vi "Read View VI and FP Refs.vi"(0 "GUI Container Actor in":refnum<class "GUI Container Actor.lvclass">, 5 "View":string, 7 "View Hierarchy Level":i32, 11 "error in (no error)":errorcluster) -> (4 "GUI Container Actor out":refnum<class "GUI Container Actor.lvclass">, 6 "View Status":T1, 8 "VI References":T4, 10 "View Found":bool, 15 "error out":errorcluster)   [LabVIEW 2023, in "GUI Views.lvlib" / "GUI Container Actor.lvclass"]
uses:
  GUI Container Actor.lvclass
  typedefs/VI References.ctl
  typedefs/View Status.ctl
  <vilib>/ActorFramework/Message Enqueuer/Message Enqueuer.lvclass
  typedefs/View Details.ctl
  typedefs/FP Status.ctl
  <userlib>/_OpenG.lib/error/error.llb/openg_error.lvlib
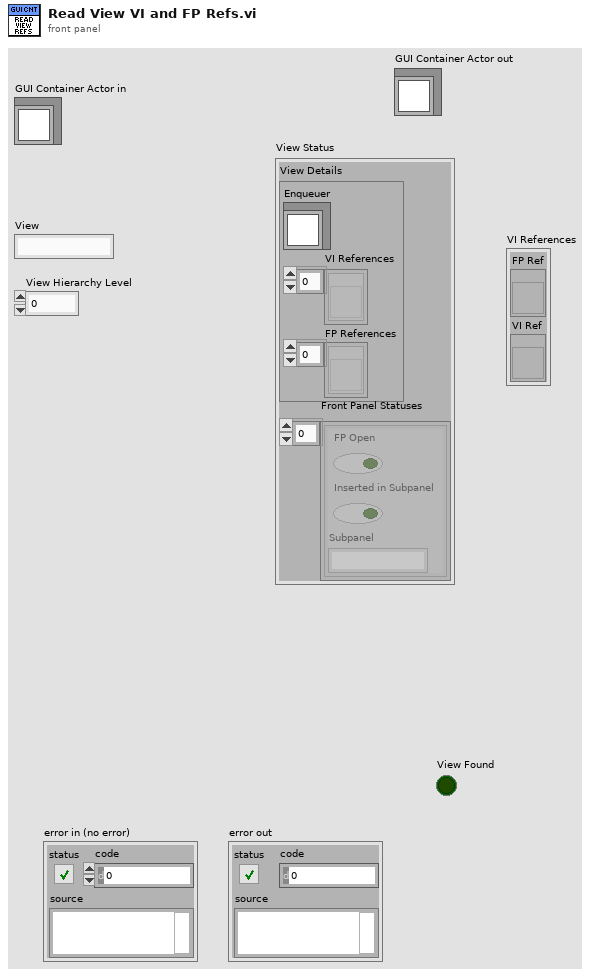
[diagram p1: front panel]
types:
  T1 = typedef "GUI Views.lvlib/GUI Container Actor.lvclass/View Status.ctl" = cluster{"View Details":T2, "Front Panel Statuses":T3[]}
  T2 = typedef "GUI Views.lvlib/GUI Container Actor.lvclass/View Details.ctl" = cluster{"Enqueuer":refnum<class "Message Enqueuer.lvclass">, "VI References":refnum<vi>[], "FP References":refnum<vi>[]}
  T3 = typedef "GUI Views.lvlib/GUI Container Actor.lvclass/FP Status.ctl" = cluster{"FP Open":bool, "Inserted in Subpanel":bool, "Subpanel":string}
  T4 = typedef "GUI Views.lvlib/GUI Container Actor.lvclass/VI References.ctl" = cluster{"FP Ref":refnum<vi>, "VI Ref":refnum<vi>}
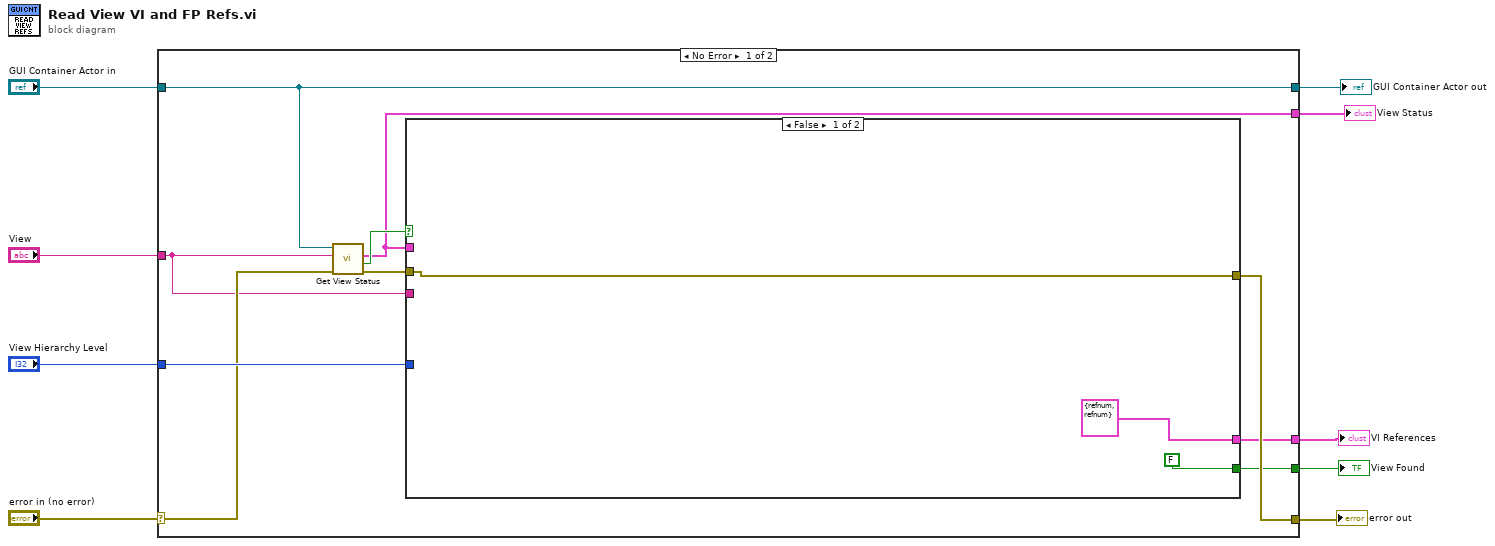
[diagram p0: block diagram]
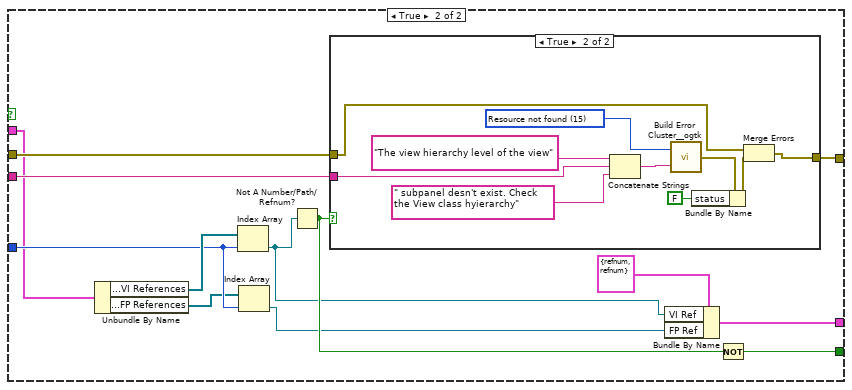
[diagram p2: hidden frame]
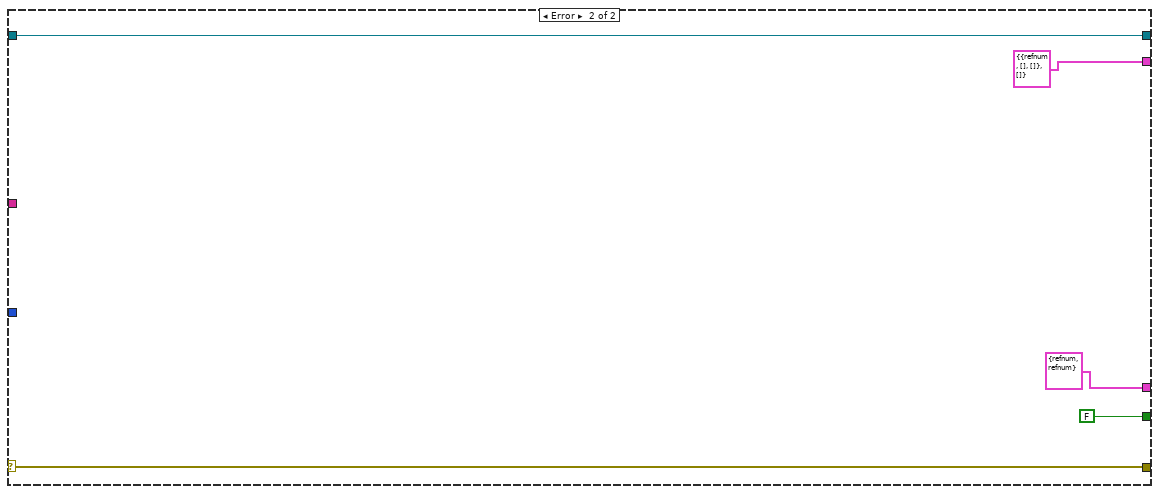
[diagram p4: hidden frame]
diagram:
  n1 = case shown="No Error" "error in (no error)" {
    selector: "error in (no error)" -> [w16 w50]
    tunnel: [w19 w50] -> w9
    tunnel: "GUI Container Actor in" -> [w13 w51]
    tunnel: "View Hierarchy Level" -> [w18 _]
    tunnel: "View" -> [w14 _]
    tunnel: [w13 w51] -> w4
    tunnel: [w17 FALSE] -> w3
    tunnel: [w11 T4 {"FP Ref"=refnum, "VI Ref"=refnum} ("VI References")] -> w2
    tunnel: [w10 T1 {"View Details"={"Enqueuer"=refnum, "VI References"=[], "FP References"=[]}, "Front Panel Statuses"=[]} ("View State")] -> w1
    frame No Error {
      n2 = call "Get View Status.vi"("error in (no error)"=w16, "View"=w14, "GUI Container View Actor in"=w13) -> ("error out"=w15:errorcluster, "View Found"=w12:bool, "View Status"=w10:T1)  [unwired: 5 in, 1 out]
      n3 = case shown="False" w12 {
        tunnel: w15 -> [w22 w34]
        tunnel: w18 -> [_ w32]
        tunnel: [w22 w33] -> w19
        tunnel: w14 -> [_ w31]
        tunnel: [FALSE w23] -> w17
        tunnel: w10 -> [_ w28]
        tunnel: [T4 {"FP Ref"=refnum, "VI Ref"=refnum} ("VI References") w24] -> w11
        frame False {
        }
        frame True {
          n4 = Unbundle By Name(w28) -> ("View Details.VI References"=w35:refnum<vi>[], "View Details.FP References"=w30:refnum<vi>[])
          n5 = Index Array(array=w35, index=w32) -> (element=w25:refnum<vi>)
          n6 = Index Array(array=w30, index=w32) -> (element=w26:refnum<vi>)
          n7 = Not A Number/Path/Refnum?(number/path/refnum=w25) -> (NaN/Path/Refnum?=w29:bool)
          n8 = case shown="True" w29 {
            tunnel: w34 -> [w36 w42]
            tunnel: [w36 w40] -> w33
            tunnel: w31 -> [_ w39]
            frame False {
            }
            frame True {
              w43 = 15 items=["No error", "Argument error", "Memory is full", "Out of zone", "End of file", "File already open", "Generic file I/O error", "File not found", "File permission error", "Disk is full", "Duplicate path", "Too many files open", "System feature not enabled", "Resource file not found", "Cannot add resource", "Resource not found", "Image not found", "Image memory error", "Pen does not exist", "Config type invalid", "Config token not found", "Config parse error", "Config memory error", "Bad external code format", "Bad external code offset", "External code not present", "Null window", "Destroy window error", "Null menu", "Print aborted", "Bad print record", "Print driver error", "Windows error during printing", "Memory error during printing", "Print dialog error", "Generic print error", "Invalid device refnum", "Device not found", "Device parameter error", "Device unit error", "Cannot open device", "Device call aborted", "Generic error", "Cancelled by user", "Object ID too low", "Object ID too high", "Object not in heap", "Unknown heap", "Unknown object (invalid DefProc)", "Unknown object (DefProc not in table)", "Message out of range", "Invalid (null) method", "Unknown message", "Manager call not supported", "Bad address", "Network operation in progress", "Network operation timed out", "Connection is busy", "Network attribute not supported", "Network error", "Address in use", "System out of memory", "Connection aborted", "Connection refused", "Not connected", "Already connected", "Connection closed", "Initialization error (interapplication manager)", "Bad occurrence", "Wait on unbound occurrence handler", "Occurrence queue overflow", "Datalog type conflict", "Unused", "Unrecognized type (interapplication manager)", "Memory corrupt", "Failed to make temporary DLL", "Old CIN version", "Drag socket not found", "Failed to load drop-object", "Failed to register OLE object", "Failed to release OLE object", "Format specifier type mismatch", "Unknown format specifier", "Too few format specifiers", "Too many format specifiers", "Scan failed", "Newer CIN version", "Error converting to variant", "Runtime menu error", "Password tampered", "Variant attribute not found", "Incompatible variant data type", "Event data is not available", "Event Store is not present", "Occurrence is not found", "Event Queue is not created", "Event info is not available", "Refnum passed is NULL", "Error retrieving Class GUID", "Error retrieving CoClass GUID", "Error retrieving TypeLib GUID.", "Bad built application magic bytes.", "Specific driver is different from the specific driver associated with the Logical Name.", "There is no session opened to the class driver.", "Max Error", "MAX - Error with config objects", "MAX - Error loading configuration", "MAX - Group not supported"]
              n9 = Concatenate Strings("The view hierarchy level of the view" ("String to Prepend to source (\"\")"), w39, " subpanel desn't exist. Check the View class hyierarchy" ("string")) -> (w45:string)
              n10 = call <userlib>:"Build Error Cluster__ogtk.vi"("String to Prepend to source (\"\")"=w45, "code"=w43) -> ("error out"=w41:errorcluster)
              n11 = Bundle By Name(cluster=w41, "status"=FALSE) -> (w38:errorcluster)
              n12 = Merge Errors(w42, w38) -> (w40:errorcluster)
            }
          }
          n13 = Bundle By Name(cluster=T4 {"FP Ref"=refnum, "VI Ref"=refnum} ("VI References"), "VI Ref"=w25, "FP Ref"=w26) -> (w24:T4)
          n14 = Not(x=w29) -> (.not. x?=w23:bool)
        }
      }
    }
    frame Error {
    }
  }
  "error out" <- w9
  "GUI Container Actor out" <- w4
  "View Found" <- w3
  "VI References" <- w2
  "View Status" <- w1
